vi "readCategoryDefaultAmount.vi"(8 "error in (no error)":errorcluster, 10 "Name":string, 11 "Account History in":refnum<class "Account History.lvclass">) -> (0 "error out":errorcluster, 2 "Default Amount":dbl, 3 "Account History out":refnum<class "Account History.lvclass">)   [LabVIEW 2020, in "Account History.lvclass"]
uses:
  Account History.lvclass
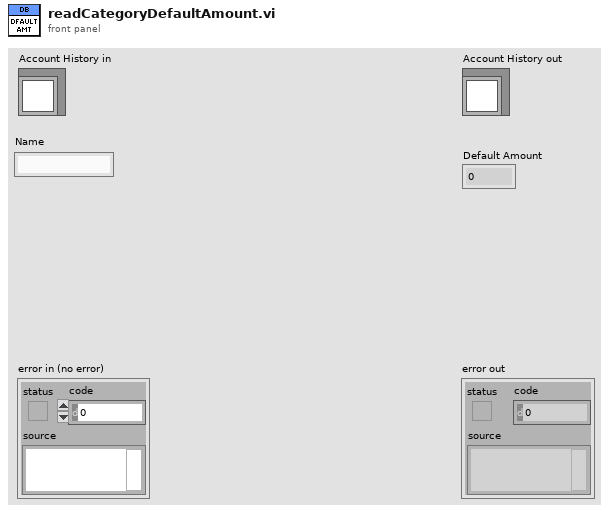
[diagram p1: front panel]
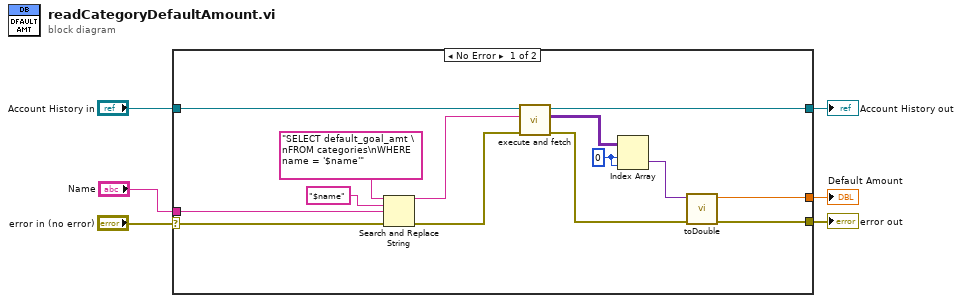
[diagram p0: block diagram]
diagram:
  n1 = case shown="No Error" "error in (no error)" {
    selector: "error in (no error)" -> [w17 w22]
    tunnel: [w8 w22] -> w5
    tunnel: [w19 w21] -> w3
    tunnel: "Account History in" -> [w20 w21]
    tunnel: "Name" -> [w12 _]
    tunnel: [w7 _] -> w1
    frame No Error {
      w11 = 0 ("index (row)")
      n2 = Search and Replace String(input string="SELECT default_goal_amt \nFROM categories\nWHERE name = '$name'", search string="$name", replace string=w12, error in=w17) -> (result string=w15:string, error out=w16:errorcluster)  [unwired: 4 in, 2 out]
      n3 = call "execute and fetch.vi"("error in (no error)"=w16, "SQL query"=w15, "Database in"=w20) -> ("error out"=w9:errorcluster, "recordset data"=w18:variant[][], "Database out"=w19:refnum<class "Account History.lvclass">)  [unwired: 6 in]
      n4 = Index Array(array=w18, index (row)=w11, index (col)=w11) -> (element=w10:variant)
      n5 = call "toDouble.vi"("error in (no error)"=w9, "Value"=w10) -> ("error out"=w8:errorcluster, "type"=w7:dbl)  [unwired: 8 in]
    }
    frame Error {
    }
  }
  "error out" <- w5
  "Account History out" <- w3
  "Default Amount" <- w1
